vi "Table_InitializeListbox.vi"(7 "This VI":refnum<vi>, 8 "error in (no error)":errorcluster, 9 "State Information":T1, 10 "Listbox Ref":refnum<vi>, 11 "NIVS.System Definition Root":refnum<k24>) -> (0 "error out":errorcluster, 1 "State Information Out":T1, 2 "Listbox Ref Out":refnum<vi>, 3 "Sorted Array out":string[][](array[string]), 5 "Limit Settings":variant)   [LabVIEW 2012, in "TableSupportLib.lvlib"]
uses:
  TableSupportLib.lvlib
  NationalInstruments.VeriStand.SystemStorage
  Table_StateInformation.ctl
  Table_ChannelInfoCluster.ctl
  Table_SortArraySettings.ctl
  Table_ListboxSettings.ctl
  NationalInstruments.VeriStand
  <userlib>/_OpenG.lib/array/array.llb/Sort 2D Array (String)__ogtk.vi
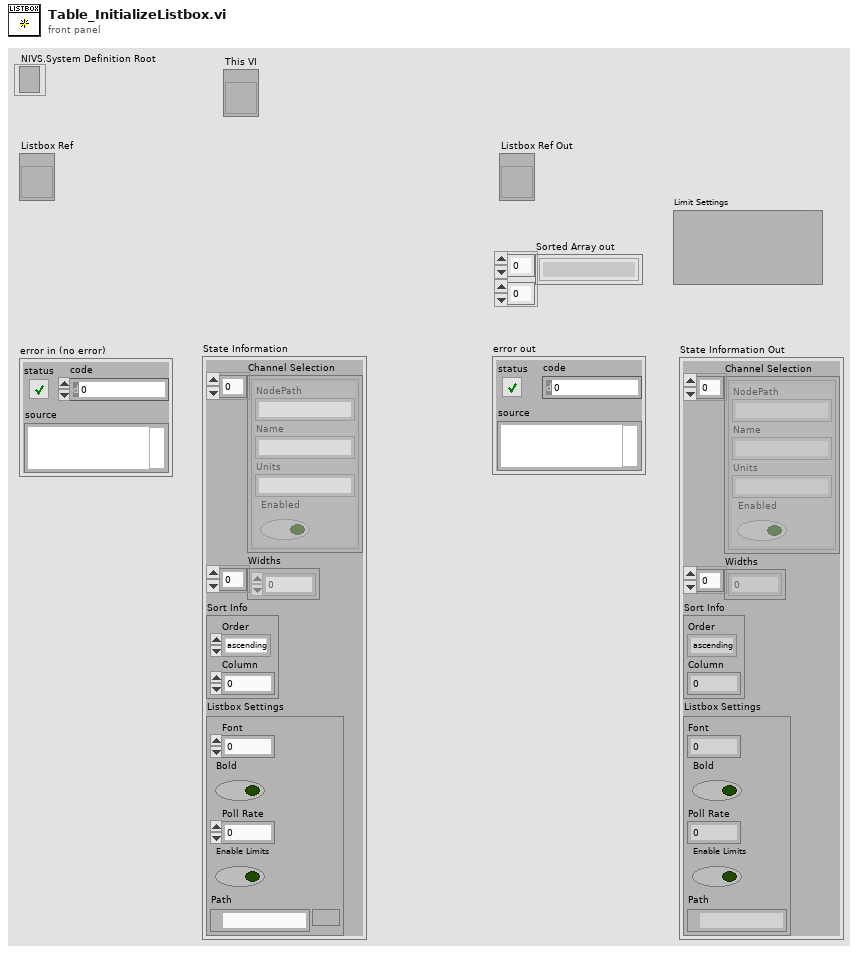
[diagram p1: front panel]
types:
  T1 = typedef "TableSupportLib.lvlib/Table_StateInformation.ctl" = cluster{"Channel Selection":T2[], "Widths":dbl[], "Sort Info":T3, "Listbox Settings":T4}
  T2 = typedef "TableSupportLib.lvlib/Table_ChannelInfoCluster.ctl" = cluster{"NodePath":string, "Name":string, "Units":string, "Enabled":bool}
  T3 = typedef "TableSupportLib.lvlib/Table_SortArraySettings.ctl" = cluster{"Order":enum16{"ascending", "descending"}, "Column":i32}
  T4 = typedef "TableSupportLib.lvlib/Table_ListboxSettings.ctl" = cluster{"Font":u32, "Bold":bool, "Poll Rate":u32, "Enable Limits":bool, "Path":path}
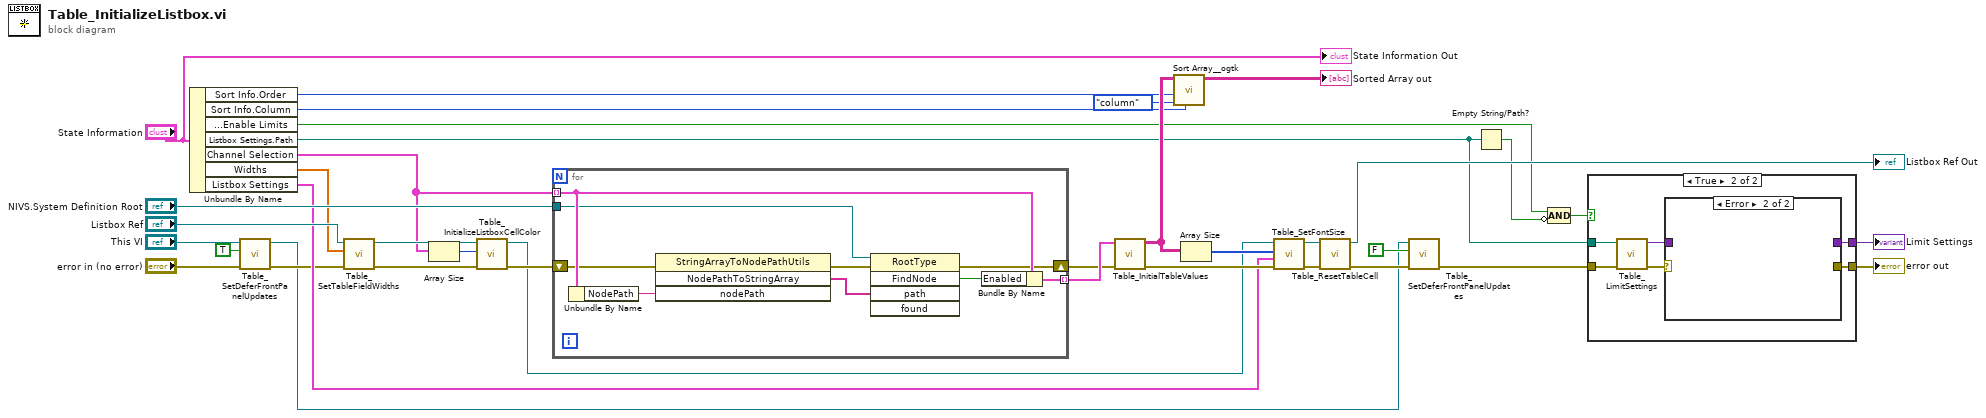
[diagram p0: block diagram]
diagram:
  n1 = Unbundle By Name("State Information") -> ("Sort Info.Order"=w34:enum16{"ascending", "descending"}, "Sort Info.Column"=w33:i32, "Listbox Settings.Enable Limits"=w10:bool, "Listbox Settings.Path"=w8:path, "Channel Selection"=w1:T2[], "Widths"=w27:dbl[], "Listbox Settings"=w24:T4)
  n2 = call "Table_SetDeferFrontPanelUpdates.vi"("error in (no error)"="error in (no error)", "Defer Panel Updates"=TRUE, "VI Ref"="This VI") -> ("error out"=w18:errorcluster, "VI Ref out"=w14:refnum<vi>)  [unwired: 7 in]
  n3 = call "Table_SetTableFieldWidths.vi"("error in (no error)"=w18, "Widths"=w27, "Listbox Ref"="Listbox Ref") -> ("error out"=w6:errorcluster, "Listbox Ref Out"=w4:refnum<vi>)  [unwired: 7 in]
  n4 = Array Size(array=w1) -> (size(s)=w2:i32)
  n5 = call "Table_InitializeListboxCellColor.vi"("error in (no error)"=w6, "Array Size"=w2, "Listbox Ref"=w4) -> ("error out"=w5:errorcluster, "Listbox Ref Out"=w3:refnum<vi>)  [unwired: 7 in]
  n6 = for {
    tunnel: w1 -> [w44] mode=indexing
    tunnel: [w42] -> w32 mode=indexing
    tunnel: "NIVS.System Definition Root" -> [w40]
    shift-right: [w38] -> w26
    shift-left: w5 -> [w39]
    n7 = Unbundle By Name(w44) -> ("NodePath"=w41:string)
    n8 = invoke class="StringArrayToNodePathUtils" method="NodePathToStringArray"(error in=w39, "nodePath"=w41) -> (error out=w45:errorcluster, "NodePathToStringArray"=w46:string[])  [unwired: 2 in, 2 out]
    n9 = invoke class="RootType" method="FindNode"(reference=w40, error in=w45, "path"=w46) -> (error out=w38:errorcluster, "FindNode"=w43:bool)  [unwired: 2 in, 3 out]
    n10 = Bundle By Name(cluster=w44, "Enabled"=w43) -> (w42:T2)
  }
  n11 = call "Table_InitialTableValues.vi"("error in"=w26, "Channel Selection"=w32) -> ("error out"=w25:errorcluster, "Table Values"=w37:string[][])  [unwired: 8 in]
  n12 = call-poly <userlib>:"Sort Array__ogtk.vi"("Column/Row to Sort By"=w33, "Sort By in"=enum16{"row", "column"}."column", "Order"=w34, "Array in"=w37) -> ("Sorted Array out"=→"Sorted Array out":string[][])  [unwired: 4 in, 3 out]
  n13 = Array Size(array=w37) -> (size(s)=w36:i32[])
  n14 = call "Table_SetFontSize.vi"("error in"=w25, "Listbox Settings"=w24, "Array Sizes"=w36, "Listbox Ref"=w3) -> ("error out"=w23:errorcluster, "Listbox Ref Out"=w22:refnum<vi>)  [unwired: 6 in]
  n15 = call "Table_ResetTableCell.vi"("error in (no error)"=w23, "Listbox Ref"=w22) -> ("error out"=w15:errorcluster, "Listbox Ref"=→"Listbox Ref Out":refnum<vi>)  [unwired: 8 in]
  n16 = call "Table_SetDeferFrontPanelUpdates.vi"("error in (no error)"=w15, "Defer Panel Updates"=FALSE, "VI Ref"=w14) -> ("error out"=w13:errorcluster)  [unwired: 7 in, 1 out]
  n17 = Empty String/Path?(string/path=w8) -> (empty?=w11:bool)
  n18 = Compound Arithmetic op=AND(w10, invert w11) -> (w9:bool)
  n19 = case shown="True" w9 {
    tunnel: w13 -> [w47 w53]
    tunnel: [w47 w50] -> w12
    tunnel: w8 -> [_ w52]
    tunnel: [_ w48] -> w7
    frame False {
    }
    frame True {
      n20 = call "Table_LimitSettings.vi"("error in"=w53, "file path (use dialog)"=w52) -> ("error out"=w51:errorcluster, "Limit Settings"=w49:variant)  [unwired: 8 in]
      n21 = case shown="Error" w51 {
        selector: w51 -> [w55 _]
        tunnel: [w55 _] -> w50
        tunnel: w49 -> [w54 _]
        tunnel: [w54 _] -> w48
        frame No Error {
        }
        frame Error {
        }
      }
    }
  }
  "error out" <- w12
  "Limit Settings" <- w7
  "State Information Out" <- "State Information"
